vi "CellArrayCell.vi"(11 "Matrix out":refnum<class "Matrix.lvclass">) -> (3 "StructEltType out":refnum<class "StructEltType.lvclass">)   [LabVIEW 2021]
uses:
  <vilib>/imath/engines/lvmath2/MathScriptCompiler/Type/Matrix.llb/Matrix.lvclass
  C:/builds/2021/dev/dist/vi.lib/imath/engines/lvmath2/MathScriptCompiler/Type.llb/Type.lvclass
  <vilib>/imath/engines/lvmath2/MathScriptCompiler/Type/StructEltType.llb/StructEltType.lvclass
  <vilib>/imath/engines/lvmath2/MathScriptCompiler/Type/StructEltType.llb/StructField.ctl
  <vilib>/imath/engines/lvmath2/MathScriptCompiler/Type.llb/Type.lvclass
  <vilib>/imath/engines/lvmath2/RunTimeEngine/Struct/NIMS_Struct_Global.vi
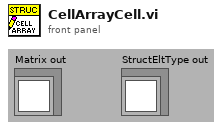
[diagram p1: front panel]
types:
  T1 = typedef "MathScriptTypes.lvlib/StructEltType.lvclass/StructField.ctl" = cluster{"Name":string, "Data Type":refnum<class "Type.lvclass">}
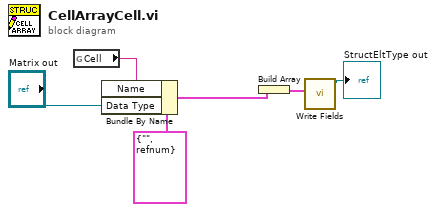
[diagram p0: block diagram]
diagram:
  n1 = global read "NIMS_Struct_Global.vi" "Cell"() -> (w6:string)
  n2 = Bundle By Name(cluster=T1 {"Name"="", "Data Type"=refnum} ("StructField"), "Name"=w6, "Data Type"="Matrix out") -> (w4:T1)
  n3 = Build Array(w4) -> (w2:T1[])
  n4 = call <vilib>:"Write Fields.vi"("Fields"=w2) -> ("StructEltType out"=→"StructEltType out":refnum<class "StructEltType.lvclass">)  [unwired: 10 in]
